vi "软件初始化.vi"   [LabVIEW 2017]
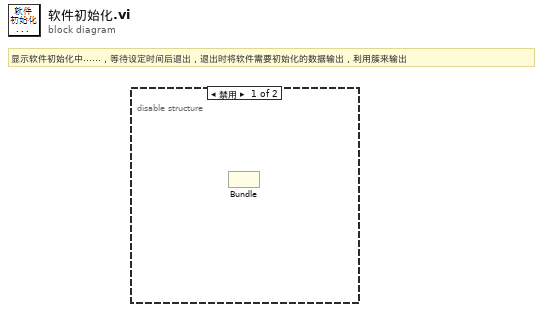
[diagram p0: block diagram]
diagram:
  # "显示软件初始化中......，等待设定时间后退出，退出时将软件需要初始化的数据输出，利用簇来输出"
  n1 = disable-structure shown="禁用" {
    frame Disabled {
      n2 = Bundle() -> ()  [unwired: 3 in, 1 out]
    }
    frame Enabled {
    }
  }
